vi "LVH5P Dset Compression and Chunking.vi"(7 "Compression Level (0-disabled)":i32, 8 "error in (no error)":errorcluster, 9 "Unlimited  dataset (F)":bool, 10 "Chunk size":u64[](array[numeric]), 11 "Dataspace Rank":u64) -> (0 "error out":errorcluster, 2 "Created dcpl?":bool, 3 "Dataset Creation Property List":T1)   [LabVIEW 2017]
uses:
  <vilib>/UPVI/lvhdf5/library.llb/HDF5 Ref.ctl
  <vilib>/UPVI/lvhdf5/property.llb/LVH5PClassId.ctl
  <vilib>/UPVI/lvhdf5/property.llb/H5D_layout_t.ctl
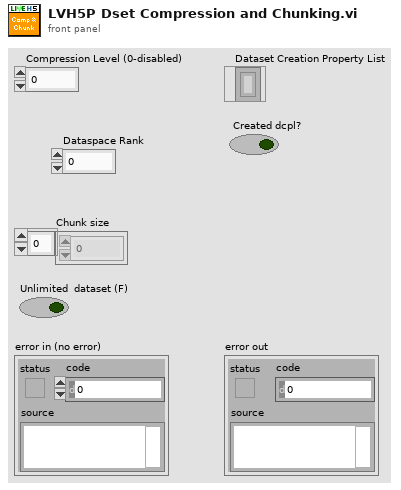
[diagram p1: front panel]
types:
  T1 = typedef "HDF5 Ref.ctl" = refnum<k1>
  T2 = typedef "LVH5PClassId.ctl" = enum32{"H5P_ROOT", "H5P_OBJECT_CREATE", "H5P_FILE_CREATE", "H5P_FILE_ACCESS", "H5P_DATASET_CREATE", "H5P_DATASET_ACCESS", "H5P_DATASET_XFER", "H5P_FILE_MOUNT", "H5P_GROUP_CREATE", "H5P_GROUP_ACCESS", "H5P_DATATYPE_CREATE", "H5P_DATATYPE_ACCESS", "H5P_STRING_CREATE", "H5P_ATTRIBUTE_CREATE", "H5P_OBJECT_COPY", "H5P_LINK_CREATE", "H5P_LINK_ACCESS"}
  T3 = typedef "H5D_layout_t.ctl" = i32
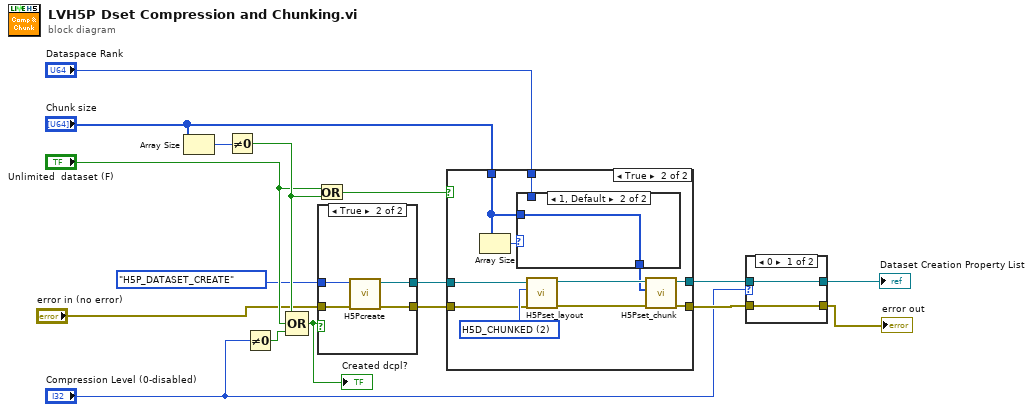
[diagram p0: block diagram]
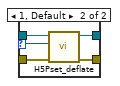
[diagram p3: hidden frame]
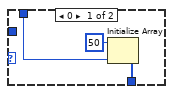
[diagram p5: hidden frame]
diagram:
  n1 = Array Size(array="Chunk size") -> (size(s)=w15:i32)
  n2 = Not Equal To 0?(x=w15) -> (x != 0?=w16:bool)
  n3 = Not Equal To 0?(x="Compression Level (0-disabled)") -> (x != 0?=w13:bool)
  n4 = Compound Arithmetic op=OR(w16, "Unlimited  dataset (F)", w13) -> (w14:bool)
  "Created dcpl?" <- w14
  n5 = Or(x="Unlimited  dataset (F)", y=w16) -> (x .or. y?=w17:bool)
  n6 = case shown="True" w14 {
    tunnel: "error in (no error)" -> [w18 w22]
    tunnel: [w18 w21] -> w11
    tunnel: [_ w20] -> w12
    tunnel: LVH5PClassId."H5P_DATASET_CREATE" ("Property List Class") -> [_ w19]
    frame False {
    }
    frame True {
      n7 = call <vilib>:"H5Pcreate.vi"("error in (no error)"=w22, "Property List Class"=w19) -> ("error out"=w21:errorcluster, "HDF5 Property List Ref"=w20:T1)  [unwired: 6 in]
    }
  }
  n8 = case shown="True" w17 {
    tunnel: w11 -> [w23 w27]
    tunnel: w12 -> [w24 w28]
    tunnel: [w24 w33] -> w7
    tunnel: [w23 w32] -> w8
    tunnel: "Dataspace Rank" -> [_ w31]
    tunnel: "Chunk size" -> [_ w26]
    frame False {
    }
    frame True {
      w35 = T3 2 items=["H5D_LAYOUT_ERROR"=-1, "H5D_COMPACT"=0, "H5D_CONTIGUOUS"=1, "H5D_CHUNKED"=2] ("Layout")
      n9 = Array Size(array=w26) -> (size(s)=w29:i32)
      n10 = case shown="1, Default" w29 {
        tunnel: w31 -> [w36 _]
        tunnel: [w37 w39] -> w30
        tunnel: w26 -> [_ w39]
        frame 0 {
          n11 = Initialize Array(50, w36) -> (w37:i32[])
        }
        frame 1, Default {
        }
      }
      n12 = call <vilib>:"H5Pset_layout.vi"("error in (no error)"=w27, "Layout"=w35, "HDF5 Property Ref"=w28) -> ("error out"=w25:errorcluster, "HDF5 Ref out"=w34:T1)  [unwired: 5 in]
      n13 = call <vilib>:"H5Pset_chunk.vi"("error in (no error)"=w25, "Dimensions"=w30, "HDF5 Property Ref"=w34) -> ("error out"=w32:errorcluster, "HDF5 Ref out"=w33:T1)  [unwired: 5 in]
    }
  }
  n14 = case shown="0" "Compression Level (0-disabled)" {
    selector: "Compression Level (0-disabled)" -> [_ w42]
    tunnel: w7 -> [w41 w46]
    tunnel: w8 -> [w40 w45]
    tunnel: [w40 w44] -> w9
    tunnel: [w41 w43] -> w10
    frame 0 {
    }
    frame 1, Default {
      n15 = call <vilib>:"H5Pset_deflate.vi"("error in (no error)"=w45, "Level (5)"=w42, "HDF5 Property Ref"=w46) -> ("error out"=w44:errorcluster, "HDF5 Ref out"=w43:T1)  [unwired: 5 in]
    }
  }
  "Dataset Creation Property List" <- w10
  "error out" <- w9
